vi "For de leds.vi"() -> ()   [LabVIEW 2016]
panel:
  out "Array 2":bool[](array[boolean])
  out "x > y?":bool
  out "Numeric Control":dbl
  in  "Array":dbl[](array[numeric])
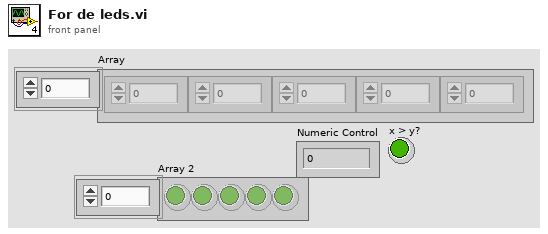
[diagram p1: front panel]
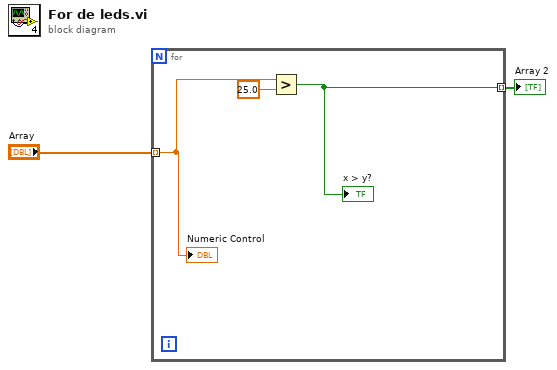
[diagram p0: block diagram]
diagram:
  n1 = for {
    tunnel: "Array" -> [w5] mode=indexing
    tunnel: [w3] -> w1 mode=indexing
    n2 = Greater?(x=w5, y=25.0) -> (0:w3:bool)
    "x > y?" <- w3
    "Numeric Control" <- w5
  }
  "Array 2" <- w1
